vi "Import File - Parse XML File.vi"(8 "error in (no error)":errorcluster, 11 "Target File":path=path "D:/Temp/UDP CD Test Files/XML Export/testExport4.xml") -> (0 "error out":errorcluster, 3 "Import/Export Data":T1 {"Tx Packets"."Tx Packet Data"."threadOptions"."pclDecimation" max=16 step=1; "Tx Packets"."Tx Packet Data"."threadOptions"."loopPeriod" max=16 step=1; "Tx Packets"."Tx Packet Data"."threadOptions"."targetPriority" min=-2 max=16 step=1; "Tx Packets"."Tx Packet Data"."threadOptions"."targetProcessor" min=-2 max=16 step=1; "Tx Packets"."Tx Packet Data"."Endianness" items=["big-endian"=0, "little-endian"=2]; "Rx Packets"."Rx Packet Data"."targetPriority" min=-2 max=16 step=1; "Rx Packets"."Rx Packet Data"."targetProcessor" min=-2 max=16 step=1; "Rx Packets"."Rx Packet Data"."Endianness" items=["big-endian"=0, "little-endian"=2]})   [LabVIEW 2016, in "UDP-Custom-Device System Explorer.lvlib"]
uses:
  UDP-Custom-Device System Explorer.lvlib
  Types/XML - New/ImpExp - Data.ctl
  Types/XML - New/ImpExp - Main Data.ctl
  <vilib>/NI Veristand/Custom Device API/Custom Device Item Info.ctl
  Types/XML - New/ImpExp - Rx Packets Data.ctl
  Types/XML - New/ImpExp - Rx Packet Data.ctl
  Shared/Types/Shared - Channel Data Type.ctl
  Shared/Types/Shared - Buffered.PacketInfo.ctl
  Shared/Types/Shared - Pointer Encoding.ctl
  Shared/Types/Shared - Receive Buffer Options.ctl
  Shared/Types/Shared - Transmit Buffer Options.ctl
  Shared/Types/Shared - New Data Options.ctl
  Types/Threading/Thread Management.ctl
  Types/XML - New/ImpExp - Tx Packets Data.ctl
  Types/XML - New/ImpExp - Tx Packet Data.ctl
  Shared/Types/Shared - Transmit Flag Options.ctl
  Shared/Types/Shared - Transmit Echo Options.ctl
  Types/Threading/Thread Configuration.ctl
  Types/Threading/Thread Sync Reference.ctl
  System.Xml
  <vilib>/NI VeriStand/Custom Device API/Custom Device API.lvlib
  Shared/UDP-Custom-Device Shared.lvlib
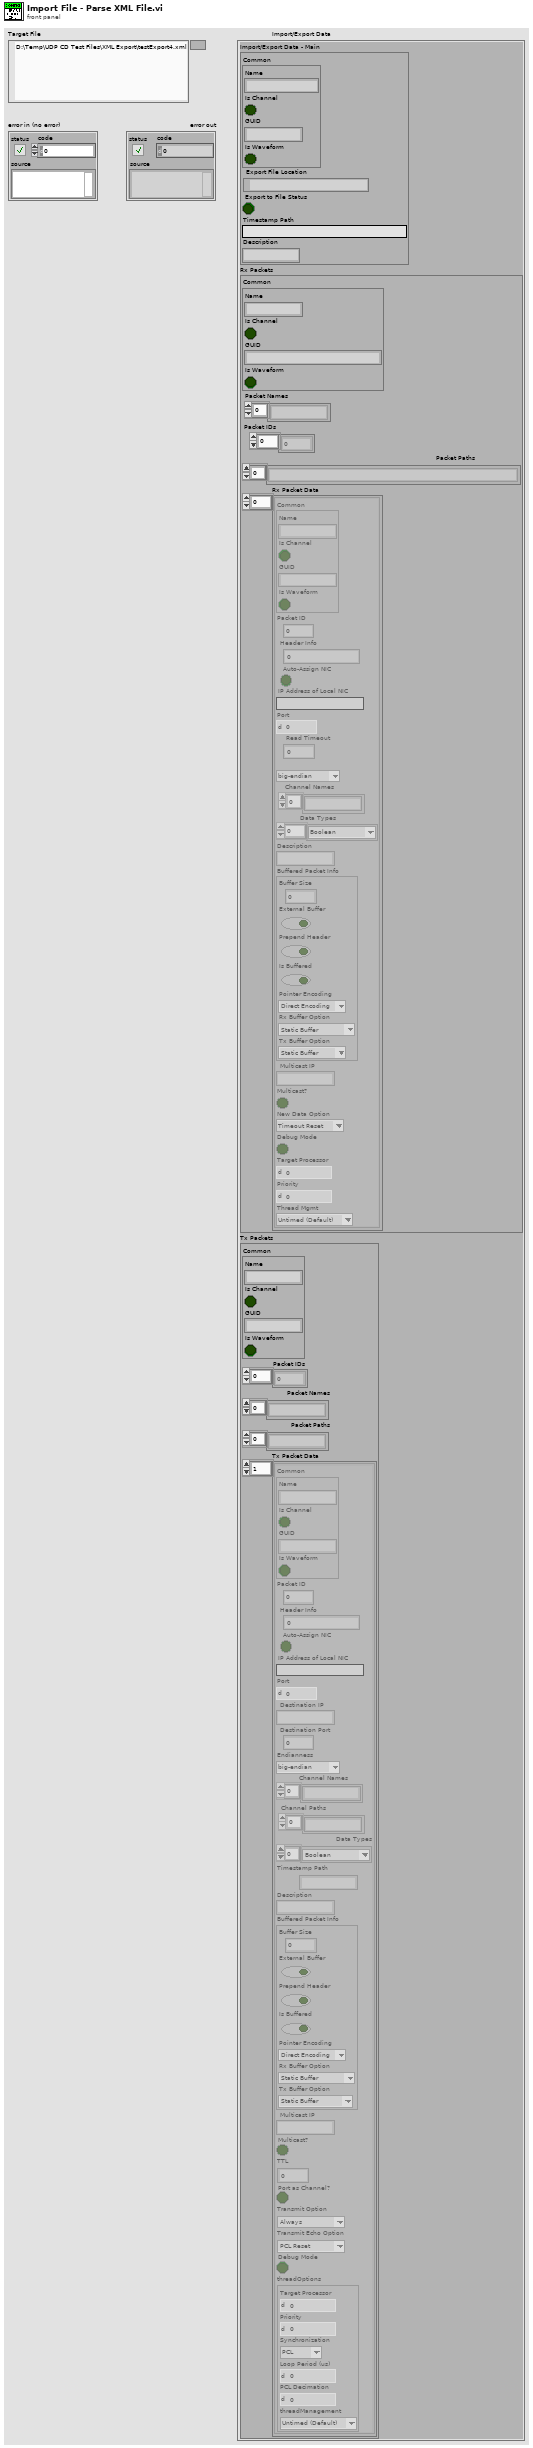
[diagram p1: front panel]
types:
  T1 = typedef "UDP-Custom-Device System Explorer.lvlib/ImpExp - Data.ctl" = cluster{"Import/Export Data - Main":T2, "Rx Packets":T4, "Tx Packets":T13}
  T2 = typedef "UDP-Custom-Device System Explorer.lvlib/ImpExp - Main Data.ctl" = cluster{"Common":T3, "Export File Location":path, "Export to File Status":bool, "Timestamp Path":string, "Description":string}
  T3 = typedef "Custom Device API.lvlib/Custom Device Item Info.ctl" = cluster{"Name":string, "Is Channel":bool, "GUID":string, "Is Waveform":bool}
  T4 = typedef "UDP-Custom-Device System Explorer.lvlib/ImpExp - Rx Packets Data.ctl" = cluster{"Common":T3, "Packet Names":string[], "Packet IDs":i32[], "Packet Paths":string[], "Rx Packet Data":T5[]}
  T5 = typedef "UDP-Custom-Device System Explorer.lvlib/ImpExp - Rx Packet Data.ctl" = cluster{"Common":T3, "Packet ID":i32, "Header Info":u32, "Auto-Assign NIC":bool, "IP Address of Local NIC":string, "Port":u16, "Read Timeout":i32, "Endianness":u16, "Channel Names":string[], "Data Types":T6[], "Description":string, "Buffered Packet Info":T7, "Multicast IP":string, "Multicast?":bool, "New Data Option":T11, "Debug Mode":bool, "targetProcessor":i8, "targetPriority":i16, "Thread Mgmt":T12}
  T6 = typedef "UDP-Custom-Device Shared.lvlib/Shared - Channel Data Type.ctl" = enum16{"Boolean", "Single", "Double", "I8", "I16", "I32", "I64", "U8", "U16", "U32", "U64"}
  T7 = typedef "UDP-Custom-Device Shared.lvlib/Shared - Buffered.PacketInfo.ctl" = cluster{"Buffer Size":i32, "External Buffer":bool, "Prepend Header":bool, "Is Buffered":bool, "Pointer Encoding":T8, "Rx Buffer Option":T9, "Tx Buffer Option":T10}
  T8 = typedef "UDP-Custom-Device Shared.lvlib/Shared - Pointer Encoding.ctl" = enum16{"Direct Encoding", "Conversion Encoding"}
  T9 = typedef "UDP-Custom-Device Shared.lvlib/Shared - Receive Buffer Options.ctl" = enum16{"Static Buffer", "Circular Buffer", "Circular Buffer + Size"}
  T10 = typedef "UDP-Custom-Device Shared.lvlib/Shared - Transmit Buffer Options.ctl" = enum16{"Static Buffer", "FIFO Buffer", "FIFO Buffer + Port"}
  T11 = typedef "UDP-Custom-Device Shared.lvlib/Shared - New Data Options.ctl" = enum16{"Timeout Reset", "Counter"}
  T12 = typedef "UDP-Custom-Device System Explorer.lvlib/Thread Management.ctl" = enum16{"Untimed (Default)", "Timed (High Priority)"}
  T13 = typedef "UDP-Custom-Device System Explorer.lvlib/ImpExp - Tx Packets Data.ctl" = cluster{"Common":T3, "Packet IDs":i32[], "Packet Names":string[], "Packet Paths":string[], "Tx Packet Data":T14[]}
  T14 = typedef "UDP-Custom-Device System Explorer.lvlib/ImpExp - Tx Packet Data.ctl" = cluster{"Common":T3, "Packet ID":i32, "Header Info":u32, "Auto-Assign NIC":bool, "IP Address of Local NIC":string, "Port":u16, "Destination IP":string, "Destination Port":u16, "Endianness":u16, "Channel Names":string[], "Channel Paths":string[], "Data Types":T6[], "Timestamp Path":string, "Description":string, "Buffered Packet Info":T7, "Multicast IP":string, "Multicast?":bool, "TTL":u16, "Port as Channel?":bool, "Transmit Option":T15, "Transmit Echo Option":T16, "Debug Mode":bool, "threadOptions":T17}
  T15 = typedef "UDP-Custom-Device Shared.lvlib/Shared - Transmit Flag Options.ctl" = enum16{"Always", "One-Shot", "Toggle"}
  T16 = typedef "UDP-Custom-Device Shared.lvlib/Shared - Transmit Echo Options.ctl" = enum16{"PCL Reset", "Counter", "Mirror"}
  T17 = typedef "UDP-Custom-Device System Explorer.lvlib/Thread Configuration.ctl" = cluster{"targetProcessor":i8, "targetPriority":i16, "Synchronization":T18, "loopPeriod":u32, "pclDecimation":u16, "threadManagement":T12}
  T18 = typedef "UDP-Custom-Device System Explorer.lvlib/Thread Sync Reference.ctl" = enum16{"PCL", "Async"}
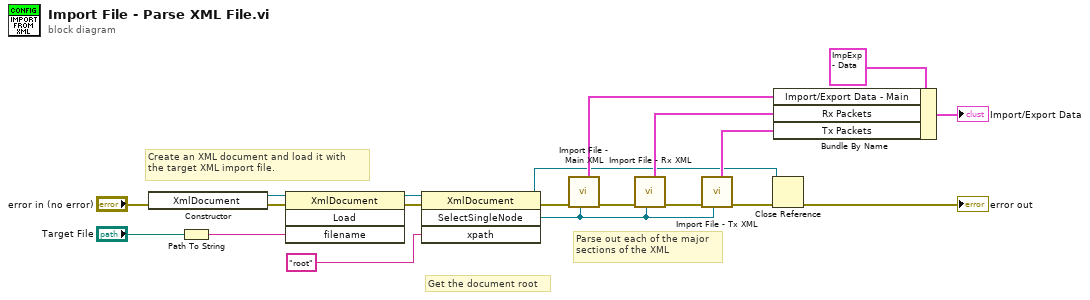
[diagram p0: block diagram]
diagram:
  # "Parse out each of the major\nsections of the XML"
  # "Get the document root"
  # "Create an XML document and load it with\nthe target XML import file."
  n1 = constructor class="XmlDocument"(error in="error in (no error)") -> (reference out=w20:refnum<k24>, error out=w19:errorcluster)  [unwired: 2 in, 1 out]
  n2 = Path To String(path="Target File") -> (string=w16:string)
  n3 = invoke class="XmlDocument" method="Load"(reference=w20, error in=w19, "filename"=w16) -> (reference out=w15:refnum<k24>, error out=w14:errorcluster)  [unwired: 1 in, 2 out]
  n4 = invoke class="XmlDocument" method="SelectSingleNode"(reference=w15, error in=w14, "xpath"="root") -> (reference out=w1:refnum<k24>, error out=w11:errorcluster, "SelectSingleNode"=w7:refnum<k24>)  [unwired: 1 in, 1 out]
  n5 = call "Import File - Main XML.vi"("Root Node"=w7, "error in (no error)"=w11) -> ("error out"=w9:errorcluster, "Main"=w2:T2)  [unwired: 8 in]
  n6 = call "Import File - Rx XML.vi"("Root Node"=w7, "error in (no error)"=w9) -> ("error out"=w10:errorcluster, "Rx Packets"=w3:T4)  [unwired: 8 in]
  n7 = call "Import File - Tx XML.vi"("Root Node"=w7, "error in (no error)"=w10) -> ("error out"=w8:errorcluster, "Tx Packets"=w4:T13)  [unwired: 8 in]
  n8 = Close Reference(reference=w1, error in (no error)=w8) -> (error out=→"error out":errorcluster)
  n9 = Bundle By Name(cluster=T1 {"Import/Export Data - Main"={"Common"={"Name"="", "Is Channel"=FALSE, "GUID"="", "Is Waveform"=FALSE}, "Export File Location"=path "", "Export to File Status"=FALSE, "Timestamp Path"="", "Description"=""}, "Rx Packets"={"Common"={"Name"="", "Is Channel"=FALSE, "GUID"="", "Is Waveform"=FALSE}, "Packet Names"=[], "Packet IDs"=[], "Packet Paths"=[], "Rx Packet Data"=[]}, "Tx Packets"={"Common"={"Name"="", "Is Channel"=FALSE, "GUID"="", "Is Waveform"=FALSE}, "Packet IDs"=[], "Packet Names"=[], "Packet Paths"=[], "Tx Packet Data"=[]}} ("Import/Export Data"), "Import/Export Data - Main"=w2, "Rx Packets"=w3, "Tx Packets"=w4) -> (→"Import/Export Data":T1)
